vi "UpdateExistingPAQtag.vi"(8 "error in (no error)":errorcluster, 10 "TAGpropertyEdit":T1 {"TAGprop"."TagFunc" format="%08x"; "TAGprop"."RangeL" format="%.2f"; "TAGprop"."RangeH" format="%.2f"}, 11 "DBAL-BIN in":refnum<class "DBAL-BIN.lvclass">) -> (0 "error out":errorcluster, 3 "DBAL-BIN out":refnum<class "DBAL-BIN.lvclass">)   [LabVIEW 2020, in "Sgraph_lib_V1.lvlib" / "DBAL-BIN.lvclass"]
doc: "Andre Koelewijn, 18 aug 2021\n\nReplace the content of one Binary TAG to the PAQprops.ini file"
uses:
  DBAL-BIN.lvclass
  controls/DBAL_TAGpropEdit.ctl
  Common/controls/typedef_com_TagProp.ctl
  DBAL-BIN.lvclass/DBAL-BIN.ctl
  <vilib>/Utility/error.llb/Error Cluster From Error Code.vi
  <vilib>/ErrorRing/Error Ring.xnode
  Builds/Sgraph_lib_V1.lvlib
  DBAL.lvclass
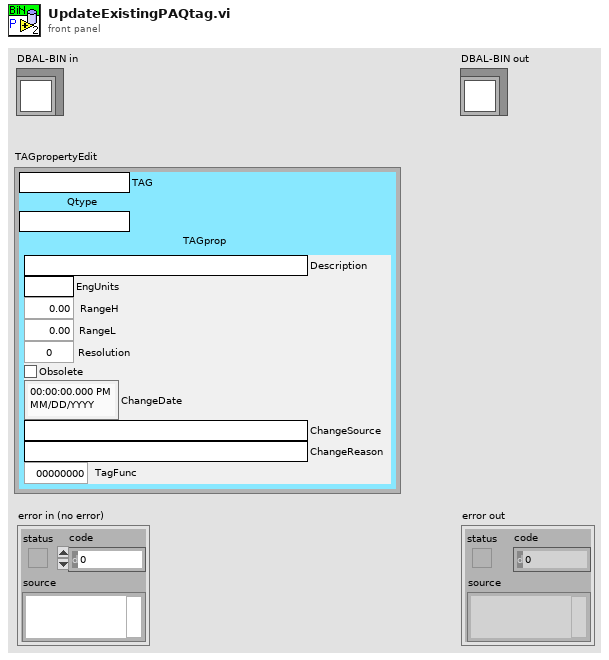
[diagram p1: front panel]
types:
  T1 = typedef "Sgraph_lib_V1.lvlib/DBAL.lvclass/DBAL_TAGpropEdit.ctl" = cluster{"TAG":string, "Qtype":string, "TAGprop":T2}
  T2 = typedef "Sgraph_lib_V1.lvlib/typedef_com_TagProp.ctl" = cluster{"Description":string, "EngUnits":string, "RangeH":dbl, "RangeL":dbl, "Resolution":i32, "Obsolete":bool, "ChangeDate":timestamp, "ChangeSource":string, "ChangeReason":string, "TagFunc":u32}
  T3 = enum16{"open", "replace", "create", "open or create", "replace or create", "replace or create with confirmation"}
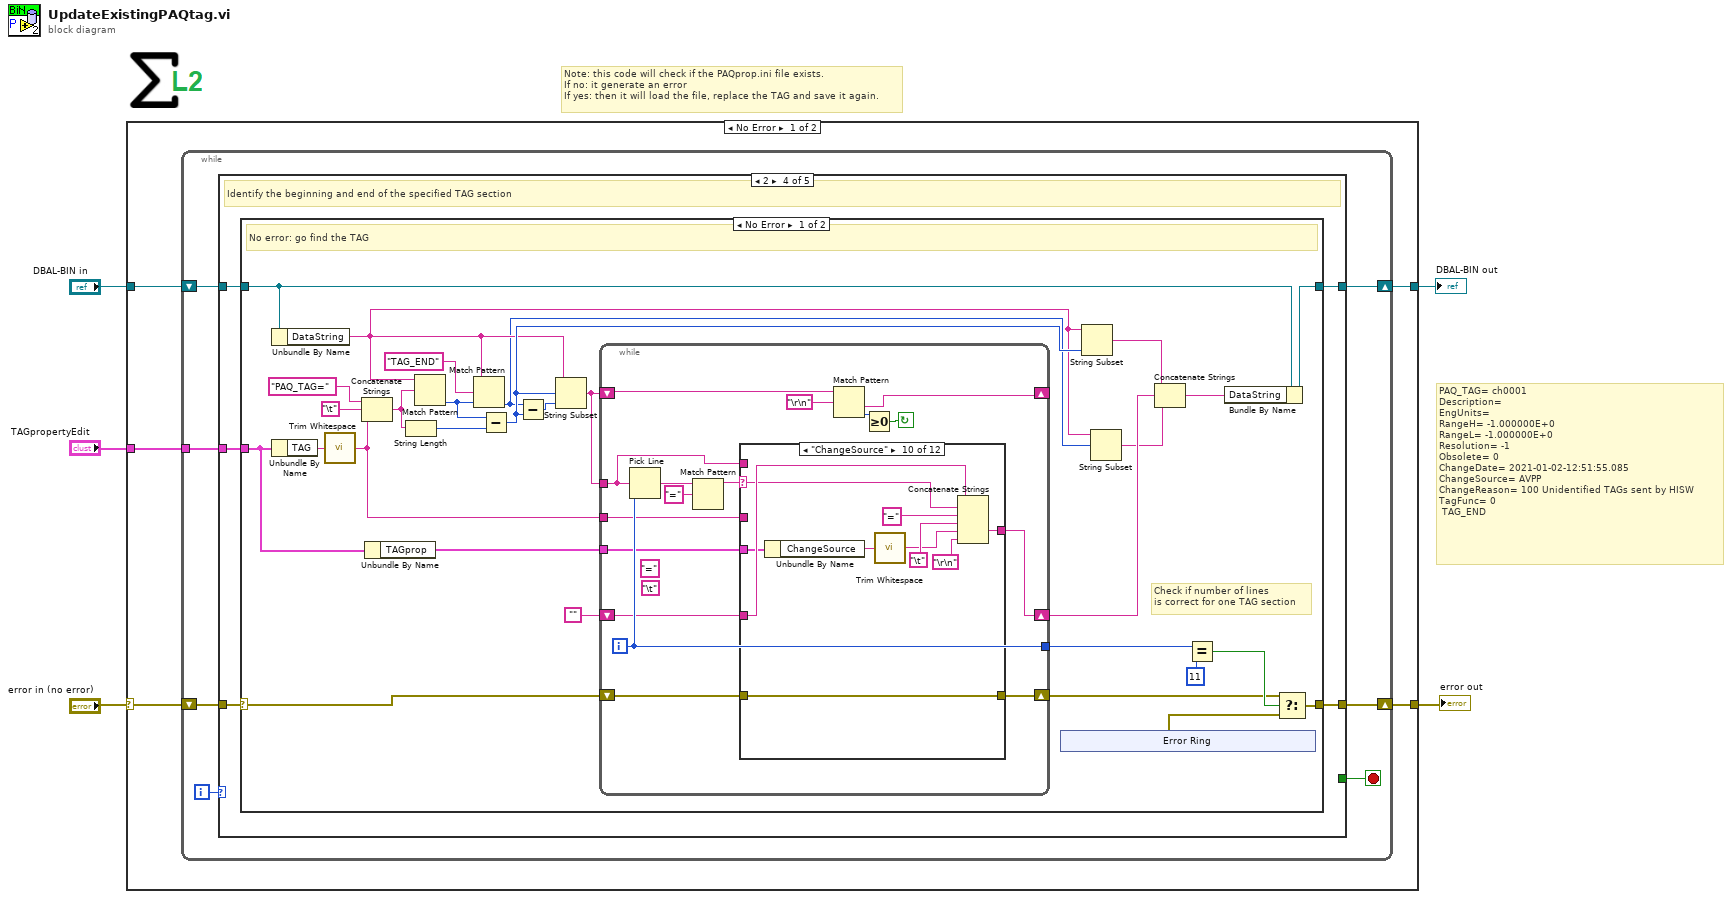
[diagram p0: block diagram]
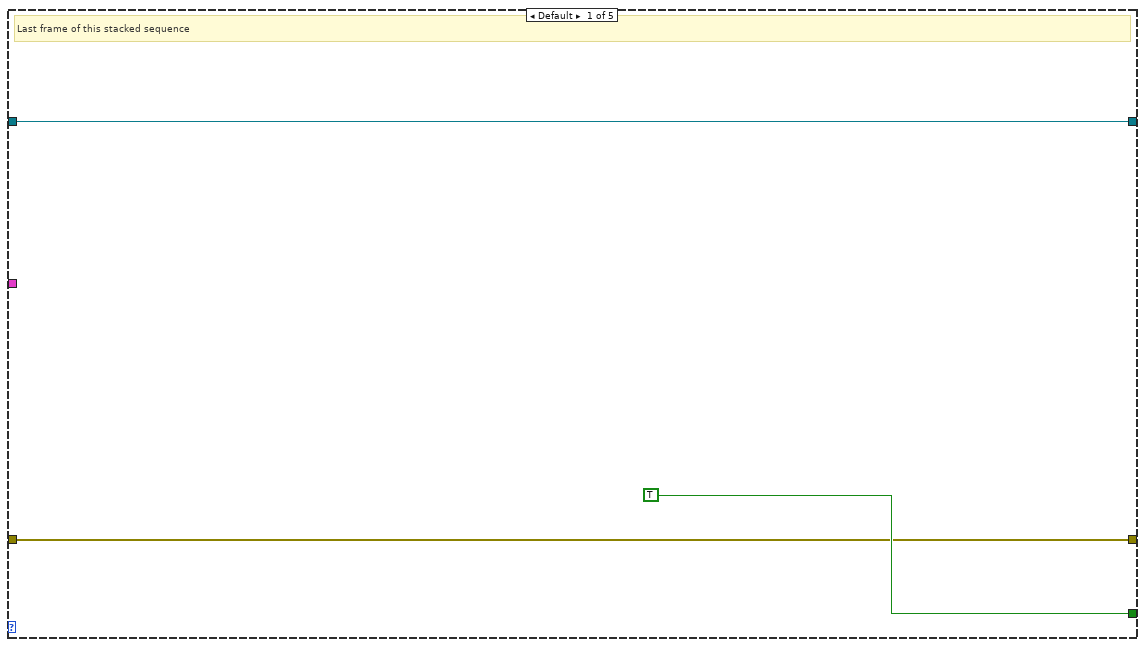
[diagram p2: hidden frame]
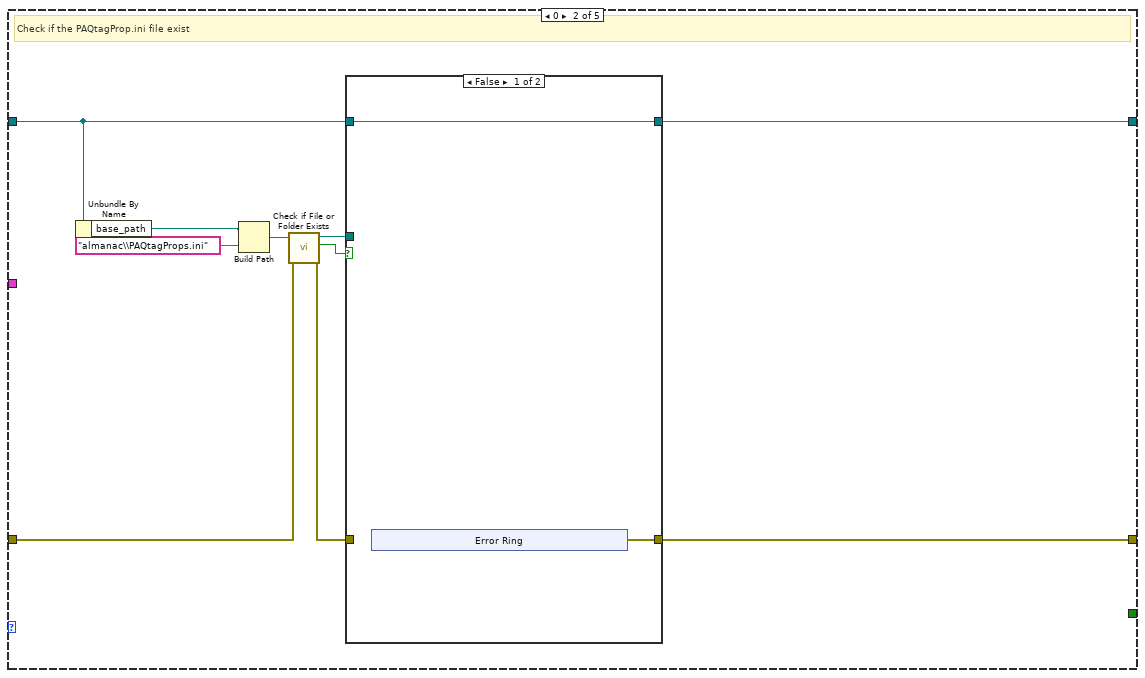
[diagram p3: hidden frame]
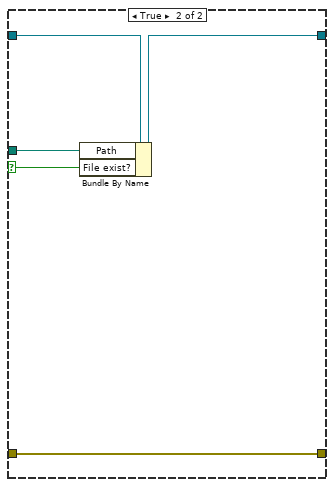
[diagram p4: hidden frame]
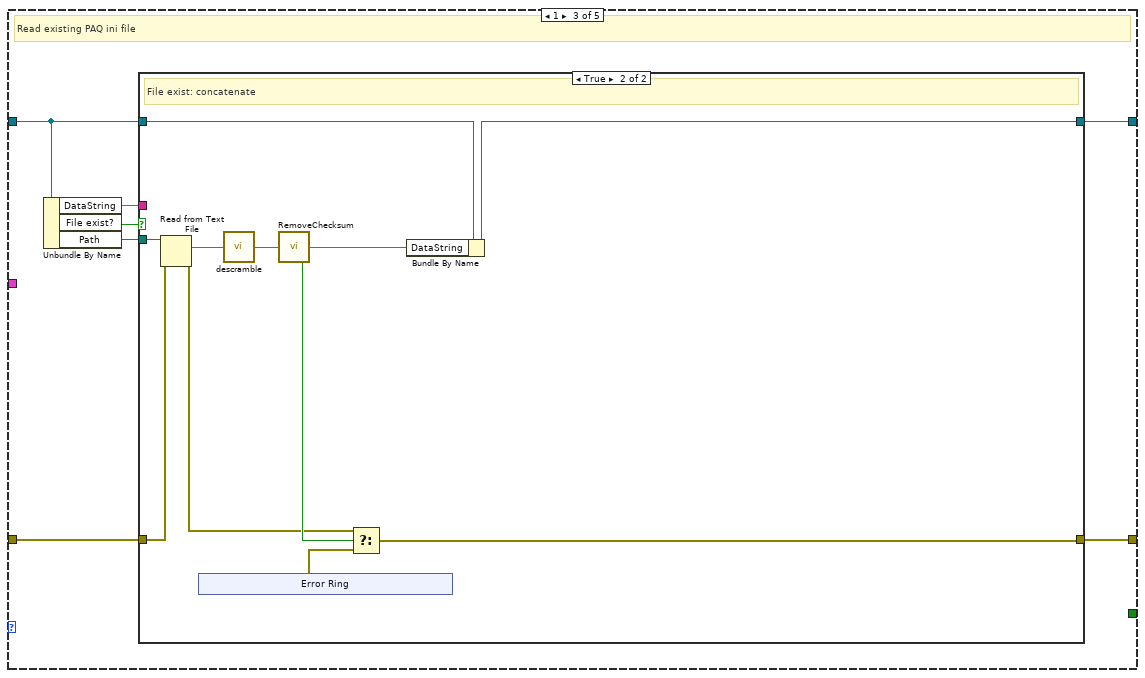
[diagram p5: hidden frame]
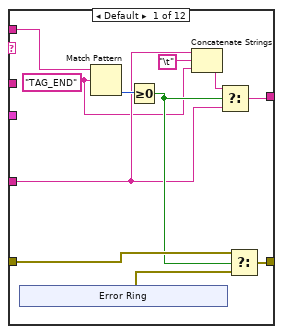
[diagram p7: hidden frame]
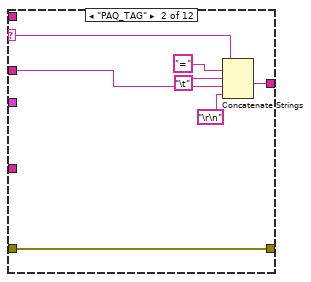
[diagram p8: hidden frame]
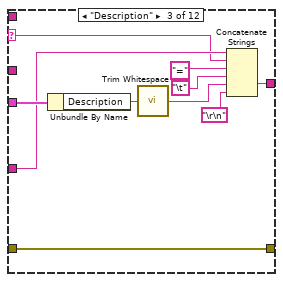
[diagram p9: hidden frame]
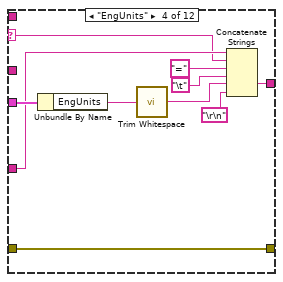
[diagram p10: hidden frame]
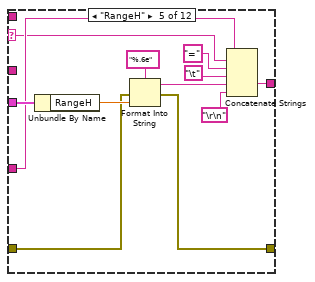
[diagram p11: hidden frame]
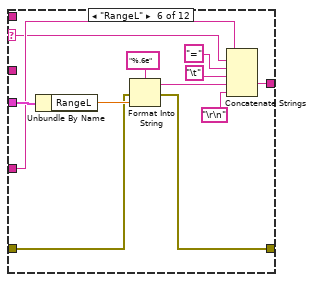
[diagram p12: hidden frame]
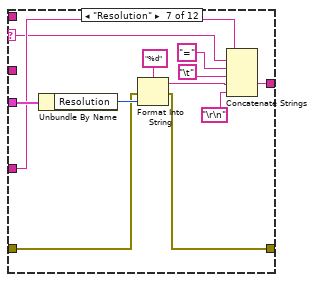
[diagram p13: hidden frame]
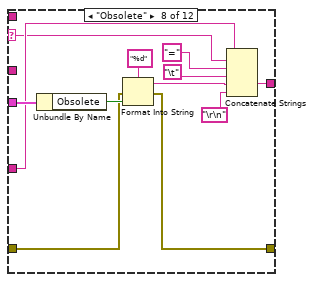
[diagram p14: hidden frame]
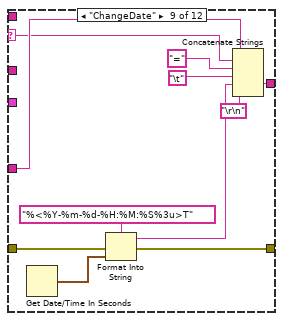
[diagram p15: hidden frame]
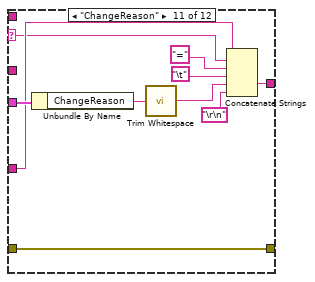
[diagram p16: hidden frame]
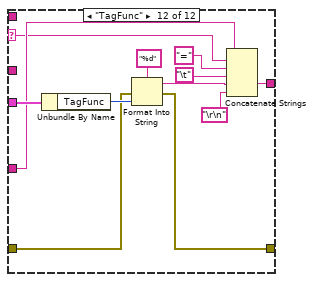
[diagram p17: hidden frame]
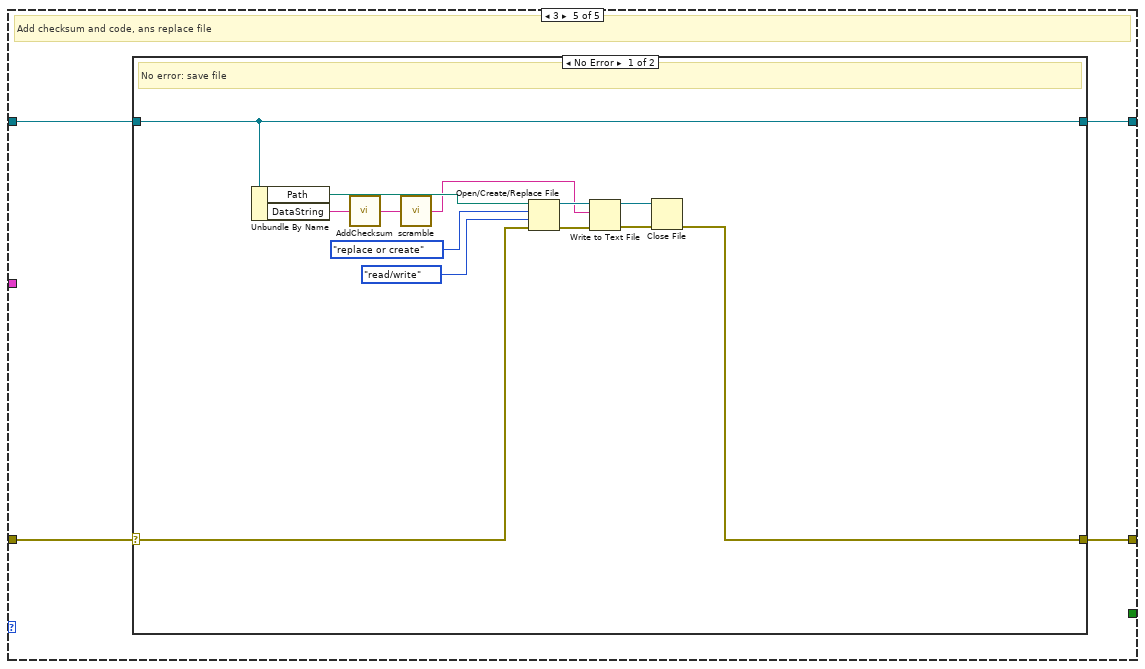
[diagram p19: hidden frame]
diagram:
  # "PAQ_TAG=\tch0001\t\nDescription=\t\t\nEngUnits=\t\t\nRangeH=\t-1.000000E+0\t\nRangeL=\t-1.000000E+0\t\nResolution=\t-1\t\nObsolete=\t0\t\nChangeDate=\t2021-01-02-12:51:55.085\t\nChangeSource=\tAVPP\t\nChangeReason=\t100 Unidentified TAGs sent by HISW\t\nTagFunc=\t0\t\n\tTAG_END"
  # "Note: this code will check if the PAQprop.ini file exists.\nIf no: it generate an error\nIf yes: then it will load the file, replace the TAG and save it again."
  n1 = case shown="No Error" "error in (no error)" {
    selector: "error in (no error)" -> [w9 w279]
    tunnel: [w7 w279] -> w2
    tunnel: [w8 w278] -> w3
    tunnel: "DBAL-BIN in" -> [w10 w278]
    tunnel: "TAGpropertyEdit" -> [w6 _]
    frame No Error {
      n2 = while {
        shift-right: [w13] -> w8
        shift-left: w10 -> [w15]
        shift-right: [w12] -> w7
        shift-left: w9 -> [w14]
        tunnel: w6 -> [w11]
        i -> [w17]
        stop <- w16 stop-if-true
        n3 = case shown="2" w17 {
          tunnel: [TRUE _ _ _ _] -> w16
          tunnel: w15 -> [w18 w24 w48 w71 w260]
          tunnel: w14 -> [w19 w28 w47 w72 w262]
          tunnel: [w18 w25 w46 w70 w259] -> w13
          tunnel: [w19 w21 w45 w69 w261] -> w12
          tunnel: w11 -> [_ _ _ w68 _]
          frame Default {
            # "Last frame of this stacked sequence"
          }
          frame 0 {
            # "Check if the PAQtagProp.ini file exist"
            n4 = Unbundle By Name(w24) -> ("base_path"=w23:path)
            n5 = Build Path(base path=w23, name or relative path="almanac\\PAQtagProps.ini") -> (appended path=w29:path)
            n6 = call <vilib>:"Check if File or Folder Exists.vi"("error in (no error)"=w28, "path"=w29) -> ("error out"=w22:errorcluster, "file or folder exists?"=w26:bool, "dup path"=w27:path)  [unwired: 7 in]
            n7 = case shown="False" w26 {
              selector: w26 -> [_ w41]
              tunnel: w27 -> [_ w42]
              tunnel: [w31 w40] -> w25
              tunnel: w24 -> [w31 w39]
              tunnel: w22 -> [_ w38]
              tunnel: [w32 w38] -> w21
              frame False {
                n8 = xnode "Error Ring"() -> ("error out"=w32:errorcluster)
              }
              frame True {
                n9 = Bundle By Name(cluster=w39, "Path"=w42, "File exist?"=w41) -> (w40:refnum<class "DBAL-BIN.lvclass">)
              }
            }
          }
          frame 1 {
            # "Read existing PAQ ini file"
            n10 = Unbundle By Name(w48) -> ("DataString"=w44:string, "File exist?"=w49:bool, "Path"=w43:path)
            n11 = case shown="True" w49 {
              tunnel: w48 -> [w51 w60]
              tunnel: w47 -> [w50 w61]
              tunnel: [w51 w59] -> w46
              tunnel: [w50 w55] -> w45
              tunnel: w44 -> [_ _]
              tunnel: w43 -> [_ w62]
              frame False {
                # "File does not exist : nothing to add"
              }
              frame True {
                # "File exist: concatenate"
                n12 = Read from Text File(file (use dialog)=w62, error in=w61) -> (text=w58:string, error out=w54:errorcluster)  [unwired: 2 in, 2 out]
                n13 = xnode "Error Ring"() -> ("error out"=w53:errorcluster)
                n14 = call "descramble.vi"("scrambled"=w58) -> ("OUT"=w57:string)  [unwired: 6 in]
                n15 = call "RemoveChecksum.vi"("IN"=w57) -> ("Check OK?"=w56:bool, "OUT"=w52:string)  [unwired: 3 in]
                n16 = Select(t=w54, s=w56, f=w53) -> (s? t:f=w55:errorcluster)
                n17 = Bundle By Name(cluster=w60, "DataString"=w52) -> (w59:refnum<class "DBAL-BIN.lvclass">)
              }
            }
          }
          frame 2 {
            # "Identify the beginning and end of the specified TAG section"
            n18 = case shown="No Error" w72 {
              selector: w72 -> [w87 w257]
              tunnel: [w91 w257] -> w69
              tunnel: w71 -> [w80 w258]
              tunnel: [w81 w258] -> w70
              tunnel: w68 -> [w85 _]
              frame No Error {
                # "Check if number of lines\nis correct for one TAG section"
                # "No error: go find the TAG"
                n19 = Unbundle By Name(w80) -> ("DataString"=w76:string)
                n20 = Unbundle By Name(w85) -> ("TAG"=w101:string)
                n21 = call <vilib>:"Trim Whitespace.vi"("string"=w101) -> ("trimmed string"=w83:string)  [unwired: 1 in]
                n22 = Concatenate Strings("PAQ_TAG=", "\t", w83) -> (w97:string)
                n23 = Unbundle By Name(w85) -> ("TAGprop"=w84:T2)
                n24 = String Length(string=w97) -> (length=w95:i32)
                n25 = Match Pattern(string=w76, regular expression=w97) -> (offset past match=w96:i32)  [unwired: 1 in, 3 out]
                n26 = Match Pattern(string=w76, regular expression="TAG_END", offset (0)=w96) -> (offset past match=w75:i32)  [unwired: 3 out]
                n27 = Subtract(x=w96, y=w95) -> (x-y=w79:i32)
                n28 = Subtract(x=w75, y=w79) -> (x-y=w94:i32)
                n29 = String Subset(string=w76, offset (0)=w79, length (rest)=w94) -> (substring=w88:string)
                n30 = while {
                  shift-right: [w121] -> _
                  shift-left: w88 -> [w122]
                  tunnel: [w117] -> w93
                  tunnel: w88 -> [w107]
                  shift-right: [w110] -> w86
                  shift-left: w87 -> [w111]
                  tunnel: w84 -> [w114]
                  tunnel: w83 -> [w113]
                  shift-right: [w108] -> w77
                  shift-left: "" -> [w112]
                  i -> [w117]
                  stop <- w118 continue-if-true
                  (unwired) "\t"
                  (unwired) "=" ("regular expression")
                  n31 = Pick Line(multi-line string=w107, line index=w117) -> (output string=w115:string)  [unwired: 1 in]
                  n32 = Match Pattern(string=w115, regular expression="=") -> (before substring=w109:string)  [unwired: 1 in, 3 out]
                  n33 = case shown="\"ChangeSource\"" w109 {
                    selector: w109 -> [_ w142 w146 w156 w166 w178 w190 w202 w214 w228 w235 w245]
                    tunnel: w114 -> [_ _ w155 w165 w177 w189 w201 w213 _ w226 w240 w256]
                    tunnel: [w127 w145 w153 w163 w175 w187 w199 w211 w223 w233 w243 w254] -> w108
                    tunnel: w113 -> [_ w139 _ _ _ _ _ _ _ _ _ _]
                    tunnel: w112 -> [w126 _ w147 w157 w167 w179 w191 w203 w215 w229 w236 w246]
                    tunnel: w111 -> [w131 w144 w150 w160 w172 w184 w196 w208 w220 w232 w242 w251]
                    tunnel: [w129 w144 w150 w160 w171 w183 w195 w207 w219 w232 w242 w250] -> w110
                    tunnel: w107 -> [w133 _ _ _ _ _ _ _ _ _ _ _]
                    frame Default {
                      w124 = "TAG_END"
                      n34 = xnode "Error Ring"() -> ("error out"=w130:errorcluster)
                      n35 = Match Pattern(string=w133, regular expression=w124) -> (offset past match=w132:i32)  [unwired: 1 in, 3 out]
                      n36 = Greater Or Equal To 0?(x=w132) -> (x >= 0?=w128:bool)
                      n37 = Concatenate Strings(w126, "\t", w124) -> (w123:string)
                      n38 = Select(t=w123, s=w128, f=w126) -> (s? t:f=w127:string)
                      n39 = Select(t=w131, s=w128, f=w130) -> (s? t:f=w129:errorcluster)
                    }
                    frame "PAQ_TAG" {
                      n40 = Concatenate Strings(w142, "=" ("regular expression"), "\t", w139, "\r\n") -> (w145:string)
                    }
                    frame "Description" {
                      n41 = Unbundle By Name(w155) -> ("Description"=w152:string)
                      n42 = call <vilib>:"Trim Whitespace.vi"("string"=w152) -> ("trimmed string"=w151:string)  [unwired: 1 in]
                      n43 = Concatenate Strings(w147, w146, "=" ("regular expression"), "\t", w151, "\r\n") -> (w153:string)
                    }
                    frame "EngUnits" {
                      n44 = Unbundle By Name(w165) -> ("EngUnits"=w162:string)
                      n45 = call <vilib>:"Trim Whitespace.vi"("string"=w162) -> ("trimmed string"=w161:string)  [unwired: 1 in]
                      n46 = Concatenate Strings(w157, w156, "=" ("regular expression"), "\t", w161, "\r\n") -> (w163:string)
                    }
                    frame "RangeH" {
                      n47 = Unbundle By Name(w177) -> ("RangeH"=w173:dbl)
                      n48 = Format Into String(format string="%.6e", error in=w172, w173) -> (resulting string=w170:string, error out=w171:errorcluster)  [unwired: 1 in]
                      n49 = Concatenate Strings(w167, w166, "=" ("regular expression"), "\t", w170, "\r\n") -> (w175:string)
                    }
                    frame "RangeL" {
                      n50 = Unbundle By Name(w189) -> ("RangeL"=w185:dbl)
                      n51 = Format Into String(format string="%.6e", error in=w184, w185) -> (resulting string=w182:string, error out=w183:errorcluster)  [unwired: 1 in]
                      n52 = Concatenate Strings(w179, w178, "=" ("regular expression"), "\t", w182, "\r\n") -> (w187:string)
                    }
                    frame "Resolution" {
                      n53 = Unbundle By Name(w201) -> ("Resolution"=w197:i32)
                      n54 = Format Into String(format string="%d", error in=w196, w197) -> (resulting string=w194:string, error out=w195:errorcluster)  [unwired: 1 in]
                      n55 = Concatenate Strings(w191, w190, "=" ("regular expression"), "\t", w194, "\r\n") -> (w199:string)
                    }
                    frame "Obsolete" {
                      n56 = Unbundle By Name(w213) -> ("Obsolete"=w209:bool)
                      n57 = Format Into String(format string="%d", error in=w208, w209) -> (resulting string=w206:string, error out=w207:errorcluster)  [unwired: 1 in]
                      n58 = Concatenate Strings(w203, w202, "=" ("regular expression"), "\t", w206, "\r\n") -> (w211:string)
                    }
                    frame "ChangeDate" {
                      n59 = Get Date/Time In Seconds() -> (seconds since 1Jan1904=w218:timestamp)
                      n60 = Format Into String(format string="%<%Y-%m-%d-%H:%M:%S%3u>T", error in=w220, w218) -> (resulting string=w221:string, error out=w219:errorcluster)  [unwired: 1 in]
                      n61 = Concatenate Strings(w215, w214, "=" ("regular expression"), "\t", w221, "\r\n") -> (w223:string)
                    }
                    frame "ChangeSource" {
                      n62 = Unbundle By Name(w226) -> ("ChangeSource"=w227:string)
                      n63 = call <vilib>:"Trim Whitespace.vi"("string"=w227) -> ("trimmed string"=w225:string)  [unwired: 1 in]
                      n64 = Concatenate Strings(w229, w228, "=" ("regular expression"), "\t", w225, "\r\n") -> (w233:string)
                    }
                    frame "ChangeReason" {
                      n65 = Unbundle By Name(w240) -> ("ChangeReason"=w241:string)
                      n66 = call <vilib>:"Trim Whitespace.vi"("string"=w241) -> ("trimmed string"=w239:string)  [unwired: 1 in]
                      n67 = Concatenate Strings(w236, w235, "=" ("regular expression"), "\t", w239, "\r\n") -> (w243:string)
                    }
                    frame "TagFunc" {
                      n68 = Unbundle By Name(w256) -> ("TagFunc"=w252:u32)
                      n69 = Format Into String(format string="%d", error in=w251, w252) -> (resulting string=w249:string, error out=w250:errorcluster)  [unwired: 1 in]
                      n70 = Concatenate Strings(w246, w245, "=" ("regular expression"), "\t", w249, "\r\n") -> (w254:string)
                    }
                  }
                  n71 = Match Pattern(string=w122, regular expression="\r\n") -> (after substring=w121:string, offset past match=w119:i32)  [unwired: 1 in, 2 out]
                  n72 = Greater Or Equal To 0?(x=w119) -> (x >= 0?=w118:bool)
                }
                n73 = xnode "Error Ring"() -> ("error out"=w89:errorcluster)
                n74 = String Subset(string=w76, length (rest)=w79) -> (substring=w78:string)  [unwired: 1 in]
                n75 = String Subset(string=w76, offset (0)=w75) -> (substring=w74:string)  [unwired: 1 in]
                n76 = Concatenate Strings(w78, w77, w74) -> (w73:string)
                n77 = Equal?(x=w93, y=11) -> (x = y?=w90:bool)
                n78 = Bundle By Name(cluster=w80, "DataString"=w73) -> (w81:refnum<class "DBAL-BIN.lvclass">)
                n79 = Select(t=w86, s=w90, f=w89) -> (s? t:f=w91:errorcluster)
              }
              frame Error {
                # "Error in the file : no action"
              }
            }
          }
          frame 3 {
            # "Add checksum and code, ans replace file"
            n80 = case shown="No Error" w262 {
              selector: w262 -> [w275 w277]
              tunnel: [w274 w277] -> w261
              tunnel: w260 -> [w263 w276]
              tunnel: [w263 w276] -> w259
              frame No Error {
                # "No error: save file"
                n81 = Unbundle By Name(w263) -> ("Path"=w271:path, "DataString"=w273:string)
                n82 = call "AddChecksum.vi"("String IN"=w273) -> ("OUT"=w272:string)  [unwired: 8 in]
                n83 = call "scramble.vi"("clean"=w272) -> ("scrambled"=w266:string)  [unwired: 6 in]
                n84 = Open/Create/Replace File(file path (use dialog)=w271, error in=w275, operation (0:open)=T3."replace or create", access (0:read/write)=enum16{"read/write", "read-only", "write-only"}."read/write") -> (refnum out=w268:refnum<file>, error out=w267:errorcluster)  [unwired: 2 in, 1 out]
                n85 = Write to Text File(file (use dialog)=w268, text=w266, error in=w267) -> (refnum out=w264:refnum<file>, error out=w265:errorcluster)  [unwired: 1 in, 1 out]
                n86 = Close File(refnum=w264, error in=w265) -> (error out=w274:errorcluster)  [unwired: 1 out]
              }
              frame Error {
                # "Error in data format: No not save file"
              }
            }
          }
        }
      }
    }
    frame Error {
    }
  }
  "error out" <- w2
  "DBAL-BIN out" <- w3
